vi "Get Variant Attribute With Defaults.vi"(9 "Variant Database defaults":variant, 10 "name":string, 11 "Variant Database from file":variant) -> (1 "values":string, 2 "found":bool, 3 "Variant out":variant)   [LabVIEW 2020]
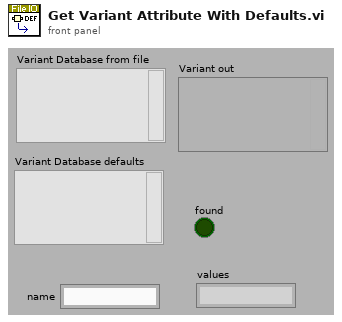
[diagram p1: front panel]
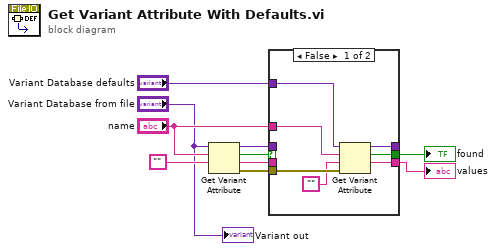
[diagram p0: block diagram]
diagram:
  n1 = Get Variant Attribute(Variant="Variant Database from file", name="name", default value (empty Variant)="") -> (duplicate Variant=w2:variant, found=w9:bool, value=w8:string, error out=w6:errorcluster)  [unwired: 1 in]
  n2 = case shown="False" w9 {
    selector: w9 -> [_ w20]
    tunnel: w8 -> [_ w19]
    tunnel: "Variant Database defaults" -> [w17 _]
    tunnel: w6 -> [w16 _]
    tunnel: "name" -> [w15 _]
    tunnel: [w14 w20] -> w4
    tunnel: [w13 w19] -> w3
    tunnel: w2 -> [_ w18]
    tunnel: [w11 w18] -> _
    frame False {
      n3 = Get Variant Attribute(Variant=w17, name=w15, default value (empty Variant)="", error in=w16) -> (duplicate Variant=w11:variant, found=w14:bool, value=w13:string)  [unwired: 1 out]
    }
    frame True {
    }
  }
  "found" <- w4
  "values" <- w3
  "Variant out" <- "Variant Database from file"
